vi "StopStreaming.vi"(8 "error in (no error)":errorcluster, 11 "CameraTestingBL in":refnum<class "CameraTesting.lvclass">) -> (0 "error out":errorcluster, 3 "CameraTestingBL out":refnum<class "CameraTesting.lvclass">)   [LabVIEW 2020, in "CameraTesting.lvlib" / "CameraTesting.lvclass"]
doc: "Send command to camera to stopping the data streaming"
uses:
  CameraTesting.lvclass
  CameraTesting.lvclass/CameraTesting.ctl
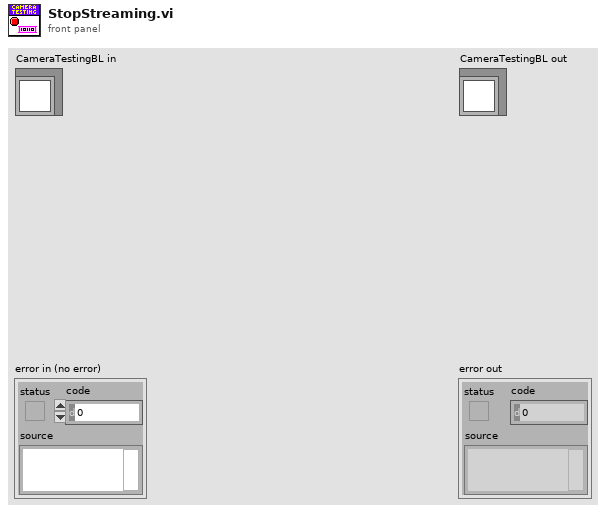
[diagram p1: front panel]
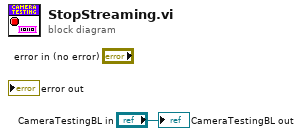
[diagram p0: block diagram]
diagram:
  "CameraTestingBL out" <- "CameraTestingBL in"
